vi "MainQueue_Analyzer.vi"(6 "timed out?":bool, 8 "error in (no error)":errorcluster, 9 "estado_queue":T1, 10 "IncioPrograma in":bool, 11 "Queue in":refnum<queue>) -> (0 "error out":errorcluster, 1 "Estado":T2, 2 "IncioPrograma out":bool, 3 "Queue out":refnum<queue>)   [LabVIEW 2026]
uses:
  Ctrl_Estados.ctl
  Control/Ctrl_DLQueue.ctl
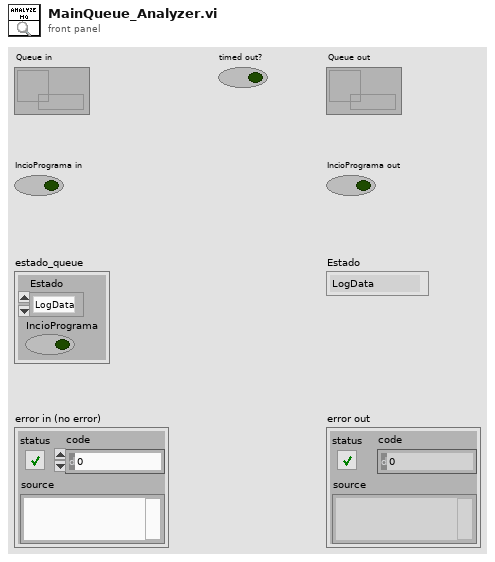
[diagram p1: front panel]
types:
  T1 = typedef "Ctrl_DLQueue.ctl" = cluster{"Estado":T2, "IncioPrograma":bool}
  T2 = typedef "Ctrl_Estados.ctl" = enum16{"LogData", "Idle", "Stop", "Log_Data_All", "Start", "HomeToHome", "Vueltas10", "Reconnect"}
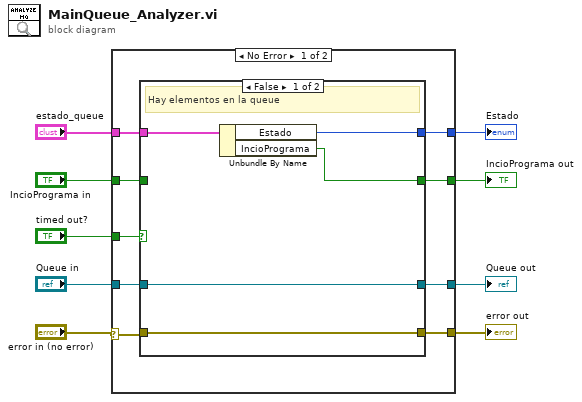
[diagram p0: block diagram]
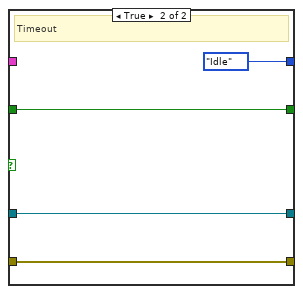
[diagram p2: hidden frame]
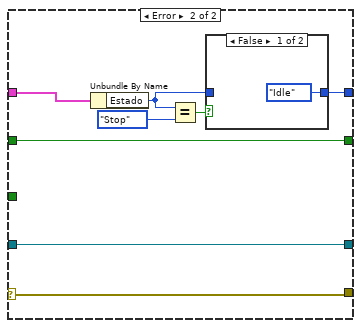
[diagram p3: hidden frame]
diagram:
  n1 = case shown="No Error" "error in (no error)" {
    selector: "error in (no error)" -> [w10 w35]
    tunnel: [w18 w29] -> w9
    tunnel: "IncioPrograma in" -> [w17 w29]
    tunnel: [w16 w30] -> w7
    tunnel: "estado_queue" -> [w15 w34]
    tunnel: "timed out?" -> [w14 _]
    tunnel: [w13 w35] -> w4
    tunnel: [w12 w28] -> w3
    tunnel: "Queue in" -> [w11 w28]
    frame No Error {
      n2 = case shown="False" w14 {
        tunnel: w11 -> [w22 w27]
        tunnel: [w22 w27] -> w12
        tunnel: w10 -> [w19 w26]
        tunnel: [w19 w26] -> w13
        tunnel: w15 -> [w23 _]
        tunnel: [w20 Ctrl_Estados."Idle" ("Estado")] -> w16
        tunnel: w17 -> [_ w25]
        tunnel: [w21 w25] -> w18
        frame False {
          # "Hay elementos en la queue"
          n3 = Unbundle By Name(w23) -> ("Estado"=w20:T2, "IncioPrograma"=w21:bool)
        }
        frame True {
          # "Timeout"
        }
      }
    }
    frame Error {
      n4 = Unbundle By Name(w34) -> ("Estado"=w31:T2)
      n5 = Equal?(x=w31, y=Ctrl_Estados."Stop") -> (x = y?=w32:bool)
      n6 = case shown="False" w32 {
        tunnel: w31 -> [_ w37]
        tunnel: [Ctrl_Estados."Idle" ("Estado") w37] -> w30
        frame False {
        }
        frame True {
        }
      }
    }
  }
  "IncioPrograma out" <- w9
  "Estado" <- w7
  "error out" <- w4
  "Queue out" <- w3
